vi "ReadAirmar.vi"(8 "Error in":errorcluster, 11 "VISA UART port":refnum<visa-resource-name>) -> (0 "Error out":errorcluster)   [LabVIEW 2013]
uses:
  <vilib>/myRIO/Instrument Drivers/Onboard IO/DIO/vis/Smart Open.vi
  <vilib>/myRIO/Instrument Drivers/Onboard IO/DIO/vis/Read.vi
  <vilib>/myRIO/Instrument Drivers/Onboard IO/DIO/vis/Open.vi
  <vilib>/myRIO/Common/Instrument Driver Framework/myRIO v1.0/DIO/vis/myRIO v1.1 Open DIO.vi
  <vilib>/myRIO/Common/Instrument Driver Framework/myRIO v1.0/DIO/vis/myRIO v1.2 Open DIO.vi
  <vilib>/myRIO/Common/Instrument Driver Framework/Utilities/vis/Validate Channels.vi
  <vilib>/myRIO/Common/Instrument Driver Framework/myRIO v1.0/DIO/vis/myRIO v1.0 Reserve DIO.vi
  <vilib>/myRIO/Common/Instrument Driver Framework/myRIO v1.0/Resource Manager/vis/myRIO v1.0 Reserve Channel List.vi
  <vilib>/myRIO/Common/Instrument Driver Framework/myRIO v1.0/DIO/vis/myRIO v1.0 Build MUX Configuration DIO.vi
  <vilib>/myRIO/Common/Instrument Driver Framework/myRIO v1.0/Resource Manager/vis/myRIO v1.0 Reserve Channel.vi
  <vilib>/myRIO/Common/Instrument Driver Framework/myRIO v1.0/Resource Manager/vis/myRIO v1.0 Unreserve Channel.vi
  <vilib>/myRIO/Common/Instrument Driver Framework/myRIO v1.0/Resource Manager/vis/myRIO v1.0 Create Configuration List.vi
  <vilib>/myRIO/Common/Instrument Driver Framework/myRIO v1.0/Resource Manager/vis/myRIO v1.0 Build Mutex Name.vi
  <vilib>/myRIO/Common/Instrument Driver Framework/Utilities/vis/Set_Get Target Info.vi
  <vilib>/Utility/error.llb/Error Cluster From Error Code.vi
  <vilib>/myRIO/Common/Instrument Driver Framework/myRIO v1.0/myRIO v1.1 Open.vi
  <vilib>/Utility/VariantDataType/GetNumericInfo.vi
  <vilib>/myRIO/Common/Instrument Driver Framework/Utilities/vis/IO Manager.vi
  <vilib>/myRIO/Common/Instrument Driver Framework/Utilities/vis/Configuration Manager.vi
  <vilib>/myRIO/Common/Instrument Driver Framework/myRIO v1.0/Resource Manager/vis/myRIO v1.0 Configure IO.vi
  <vilib>/myRIO/Common/Instrument Driver Framework/myRIO v1.0/myRIO v1.0 Close.vi
  <vilib>/myRIO/Common/Instrument Driver Framework/myRIO v1.0/myRIO v1.2 Open.vi
  <vilib>/myRIO/Common/Instrument Driver Framework/myRIO v1.0/DIO/vis/myRIO v1.0 Read DIO.vi
panel:
  out "Longitude [deg]":string
  out "Latitude [deg]":string
  in  "time zone":i32
  out "Time":string
  out "Mode":string
  out "Date [ddmmyy]":string
  out "Course over ground [degrees]":string
  out "Status":string
  out "Speed over ground [knots]":string
  out "E/W":string
  out "Longitude":string
  out "N/S":string
  out "Latitude":string
  out "UTC Time":string
  out "1PPS":bool
  out "NMEA sentences":string
  # "GPS demo"
  # "[hhmmss.sss]"
  # "A = vAlid data\nV = inValid data"
  # "[ddmm.mmmm]"
  # "[dddmm.mmmm]"
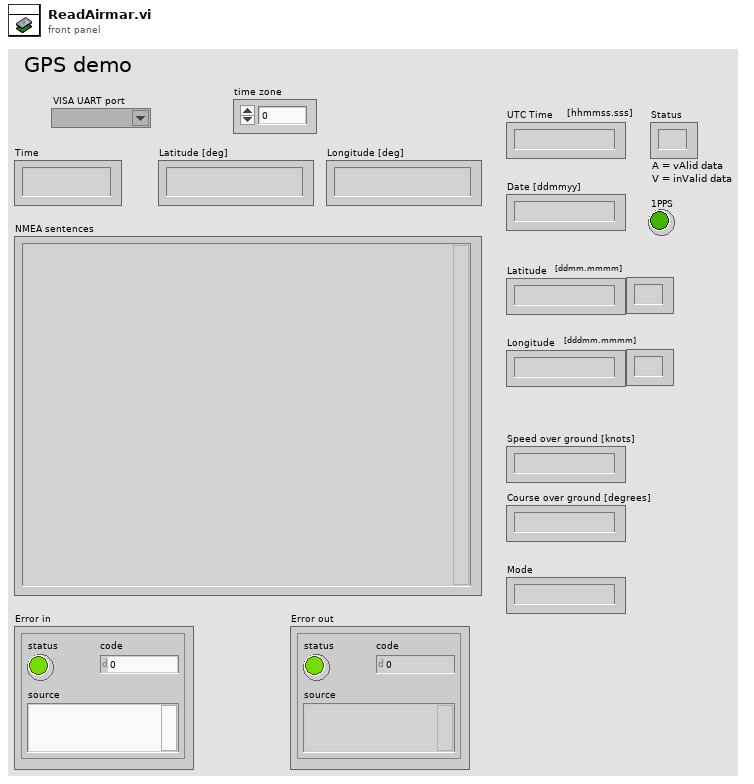
[diagram p1: front panel]
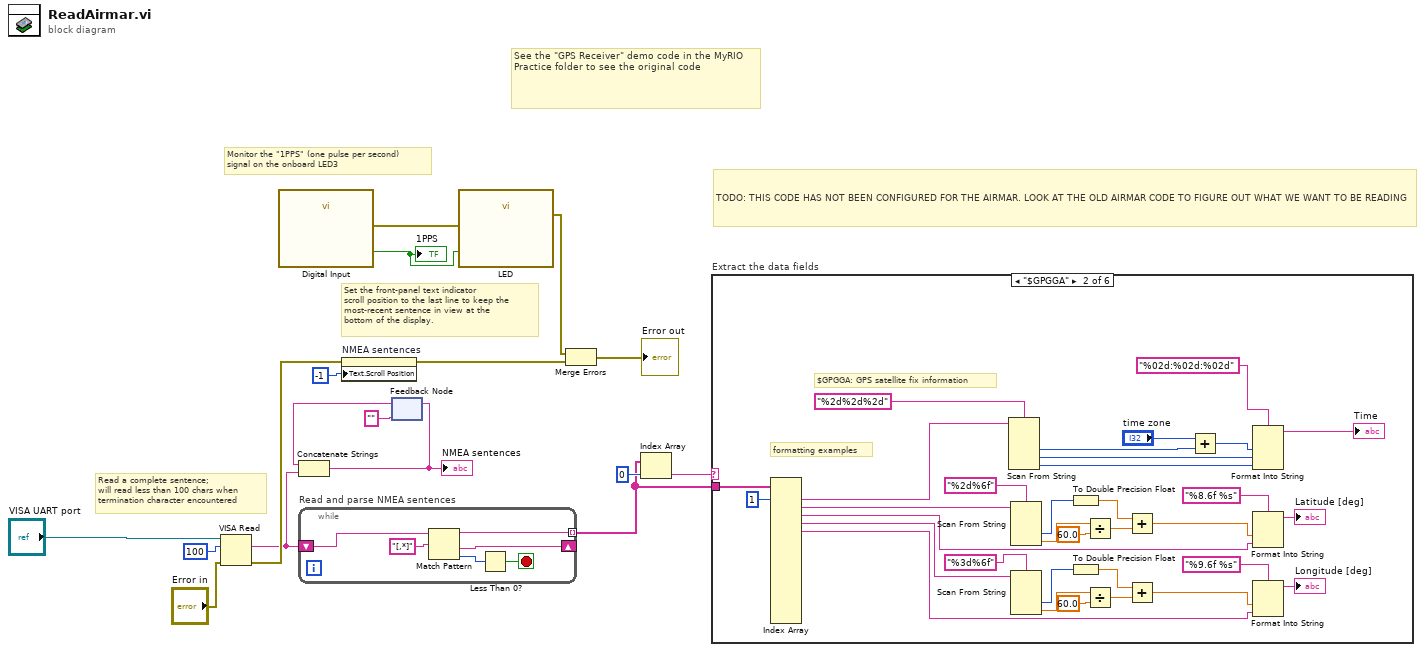
[diagram p0: block diagram]
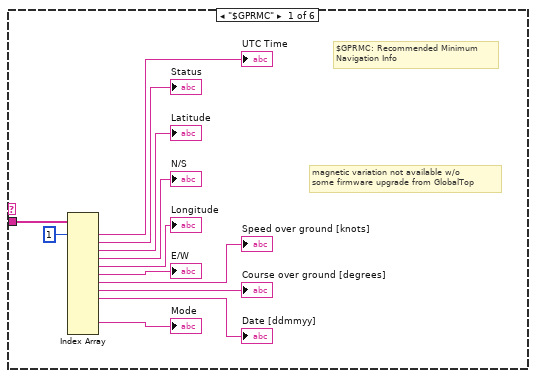
[diagram p2: hidden frame]
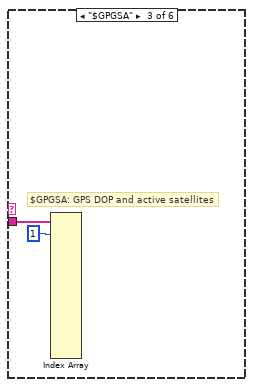
[diagram p3: hidden frame]
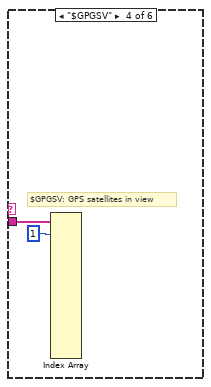
[diagram p4: hidden frame]
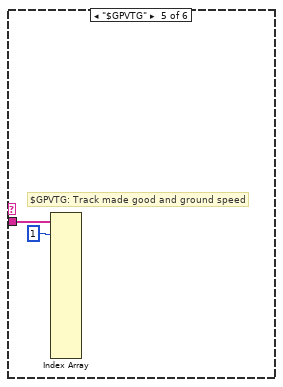
[diagram p5: hidden frame]
diagram:
  # "TODO: THIS CODE HAS NOT BEEN CONFIGURED FOR THE AIRMAR. LOOK AT THE OLD AIRMAR CODE TO FIGURE OUT WHAT WE WANT TO BE READING"
  # "Set the front-panel text indicator\nscroll position to the last line to keep the\nmost-recent sentence in view at the\nbottom of the display."
  # "Read a complete sentence;\nwill read less than 100 chars when\ntermination character encountered"
  # "Monitor the \"1PPS\" (one pulse per second)\nsignal on the onboard LED3"
  # "See the \"GPS Receiver\" demo code in the MyRIO Practice folder to see the original code"
  n1 = VISA Read(VISA resource name="VISA UART port", byte count=u32 100, error in (no error)="Error in") -> (read buffer=w8:string, error out=w13:errorcluster)  [unwired: 2 out]
  n2 = call "Digital Input"() -> ("A/DIO0 (Pin 11)"=w15:bool, "error out"=w16:errorcluster)  [unwired: 26 in]
  "1PPS" <- w15
  n3 = while "Read and parse NMEA sentences" {
    tunnel: [w21] -> w10 mode=indexing
    shift-right: [w20] -> _
    shift-left: w8 -> [w22]
    stop <- w19 stop-if-true
    n4 = Match Pattern(string=w22, regular expression="[,*]") -> (before substring=w21:string, after substring=w20:string, offset past match=w18:i32)  [unwired: 1 in, 1 out]
    n5 = Less Than 0?(x=w18) -> (x < 0?=w19:bool)
  }
  n6 = property on="NMEA sentences" class="Str"(error in=w13, "Text.Scroll Position"=-1) -> (error out=w1:errorcluster)  [unwired: 1 in, 1 out]
  n7 = feedback #1("") -> (w6:string)
  n8 = Concatenate Strings "Concatenate Strings"(w6, w8) -> (w4:string)
  "NMEA sentences" <- w4
  n9 = feedback-in #1(w4) -> ()
  n10 = call "LED"("LED3"=w15, "error in (no error)"=w16) -> ("error out"=w14:errorcluster)  [unwired: 25 in]
  n11 = Merge Errors "Merge Errors"(w14, w1) -> (→"Error out":errorcluster)
  n12 = Index Array "Index Array"(array=w10, index=0) -> (element=w9:string)
  n13 = case "Extract the data fields" shown="\"$GPGGA\"" w9 {
    tunnel: w10 -> [w35 w68 w70 w72 w74 _]
    frame "$GPRMC" {
      # "magnetic variation not available w/o\nsome firmware upgrade from GlobalTop"
      # "$GPRMC: Recommended Minimum\nNavigation Info"
      n14 = Index Array "Index Array"(array=w35, index #1=1 ("index")) -> (element #1=→"UTC Time":string, element #2=→"Status":string, element #3=→"Latitude":string, element #4=→"N/S":string, element #5=→"Longitude":string, element #6=→"E/W":string, element #7=→"Speed over ground [knots]":string, element #8=→"Course over ground [degrees]":string, element #9=→"Date [ddmmyy]":string, element #12=→"Mode":string)  [unwired: 12 in, 3 out]
    }
    frame "$GPGGA" {
      # "formatting examples"
      # "$GPGGA: GPS satellite fix information"
      n15 = Index Array "Index Array"(array=w68, index #1=1 ("index")) -> (element #1=w65:string, element #2=w56:string, element #3=w48:string, element #4=w37:string, element #5=w36:string)  [unwired: 15 in, 11 out]
      n16 = Scan From String "Scan From String"(format string="%2d%2d%2d", input string=w65) -> (output 1=w58:i32, output 2=w61:i32, output 3=w63:i32)  [unwired: 5 in, 3 out]
      n17 = Scan From String(format string="%2d%6f", input string=w56) -> (output 1=w53:i32, output 2=w55:dbl)  [unwired: 4 in, 3 out]
      n18 = Scan From String(format string="%3d%6f", input string=w37) -> (output 1=w41:i32, output 2=w39:dbl)  [unwired: 4 in, 3 out]
      n19 = To Double Precision Float(number=w53) -> (double precision float=w51:dbl)
      n20 = To Double Precision Float(number=w41) -> (double precision float=w43:dbl)
      n21 = Divide(x=w55, y=60.0) -> (x/y=w52:dbl)
      n22 = Divide(x=w39, y=60.0) -> (x/y=w42:dbl)
      n23 = Add(x=w51, y=w52) -> (x+y=w49:dbl)
      n24 = Add(x=w43, y=w42) -> (x+y=w45:dbl)
      n25 = Add(x="time zone", y=w58) -> (x+y=w59:i32)
      n26 = Format Into String "Format Into String"(format string="%02d:%02d:%02d", w59, w61, w63) -> (resulting string=→"Time":string)  [unwired: 2 in, 1 out]
      n27 = Format Into String(format string="%8.6f %s", w49, w48) -> (resulting string=→"Latitude [deg]":string)  [unwired: 2 in, 1 out]
      n28 = Format Into String(format string="%9.6f %s", w45, w36) -> (resulting string=→"Longitude [deg]":string)  [unwired: 2 in, 1 out]
    }
    frame "$GPGSA" {
      # "$GPGSA: GPS DOP and active satellites"
      n29 = Index Array(array=w70, index #1=1 ("index")) -> ()  [unwired: 15 in, 16 out]
    }
    frame "$GPGSV" {
      # "$GPGSV: GPS satellites in view"
      n30 = Index Array(array=w72, index #1=1 ("index")) -> ()  [unwired: 15 in, 16 out]
    }
    frame "$GPVTG" {
      # "$GPVTG: Track made good and ground speed"
      n31 = Index Array(array=w74, index #1=1 ("index")) -> ()  [unwired: 15 in, 16 out]
    }
    frame Default {
    }
  }
